vi "GUI_PR4000_flow.vi"() -> ()   [LabVIEW 2013]
uses:
  Shared/GUI_Template/GUI_master/tcp_new_data_event.ctl
  Shared/GUI_Template/GUI_master/tcp new data cluster.ctl
  controlFGV_TYPDEF.ctl
panel:
  in  "SlaveValue::1":dbl=25.5 caption="Slave value (%)" min=0.0 max=100.0 format="%_4f"
  in  "slaveenable::1":bool caption="Slave Mode"
  in  "Data.Channel 2::1":dbl=25.5 caption="PR4000 Pressure 2" min=0.0 max=1000.0 format="%_4f"
  out "Data.Channel 2::3":dbl=25.5 caption="PR4000 Flow 2" min=0.0 max=1000.0 format="%_4f"
  in  "Tab Control":enum32{"Chart", "Devices"}(tab)
  out "XY Graph":cluster{dbl[], dbl[]}[](graph)
  in  "Auto-scale horizontal range":bool caption="Force selected range"
  in  "Range graph3 (hours) 2":dbl=3.0 caption="Range (hours)"
  in  "Clear":bool
  in  "GUIdevice 2":string="BELLA_PDR2000"
  in  "GUIdevice 1":string="PL1-PresCtrl-Low1"
  in  "GUIdevice 3":string="PL1-PresCtrl-Low2"
  out "pressure2::2":dbl=25.5 caption="PDR pressure 2" min=-100.0 max=500.0 format="%_4f"
  out "Data.Channel 1::3":dbl=25.5 caption="PR4000 Flow 1" min=0.0 max=1000.0 format="%_4f"
  in  "Data.Channel 1::1":dbl=25.5 caption="PR4000 Pressure 1" min=0.0 max=1000.0 format="%_4f"
  out "pressure::2":dbl=25.5 caption="PDR Pressure 1" min=-100.0 max=500.0 format="%_4f"
  out "error IO 2":errorcluster
  in  "insert tag":bool=TRUE
  out "tcp data event":T1
  in  "stop":bool
  in  "UDP error message":string
  # "Plasma 1 capillary pressure & flow"
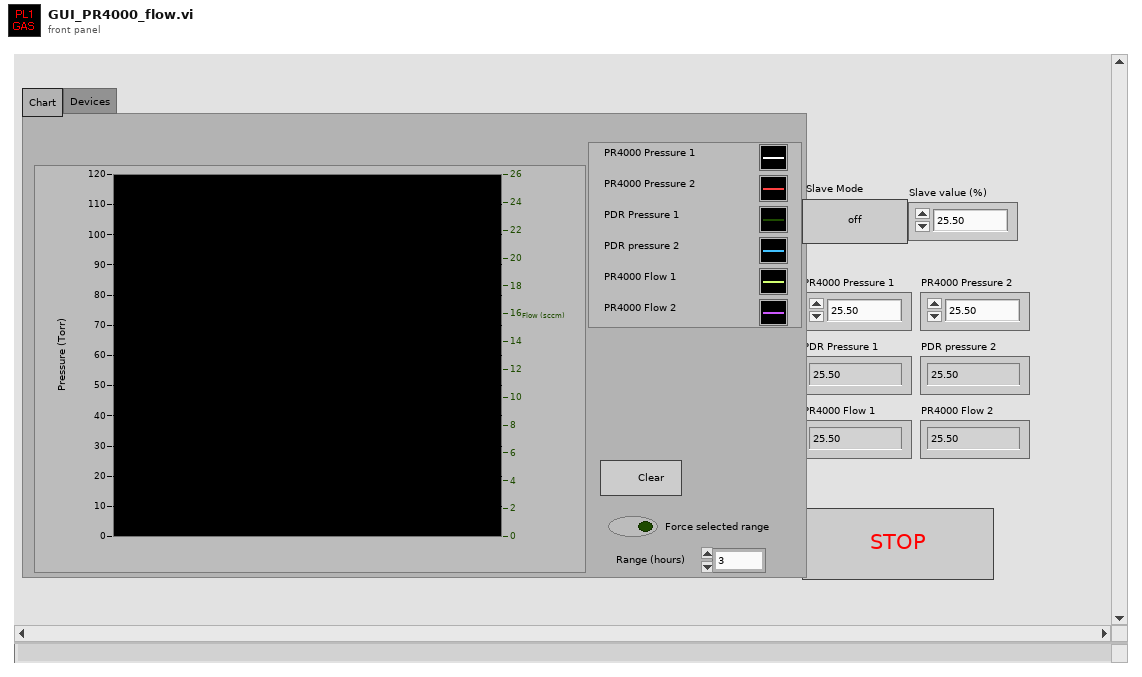
[diagram p1: front panel]
types:
  T1 = typedef "tcp_new_data_event.ctl" = refnum<user-event>
  T2 = typedef "tcp new data cluster.ctl" = cluster{"EventEnum":enum16{"new data", "connection status update"}, "Device name":string}
  T3 = typedef "controlFGV_TYPDEF.ctl" = enum16{"read", "write", "clear"}
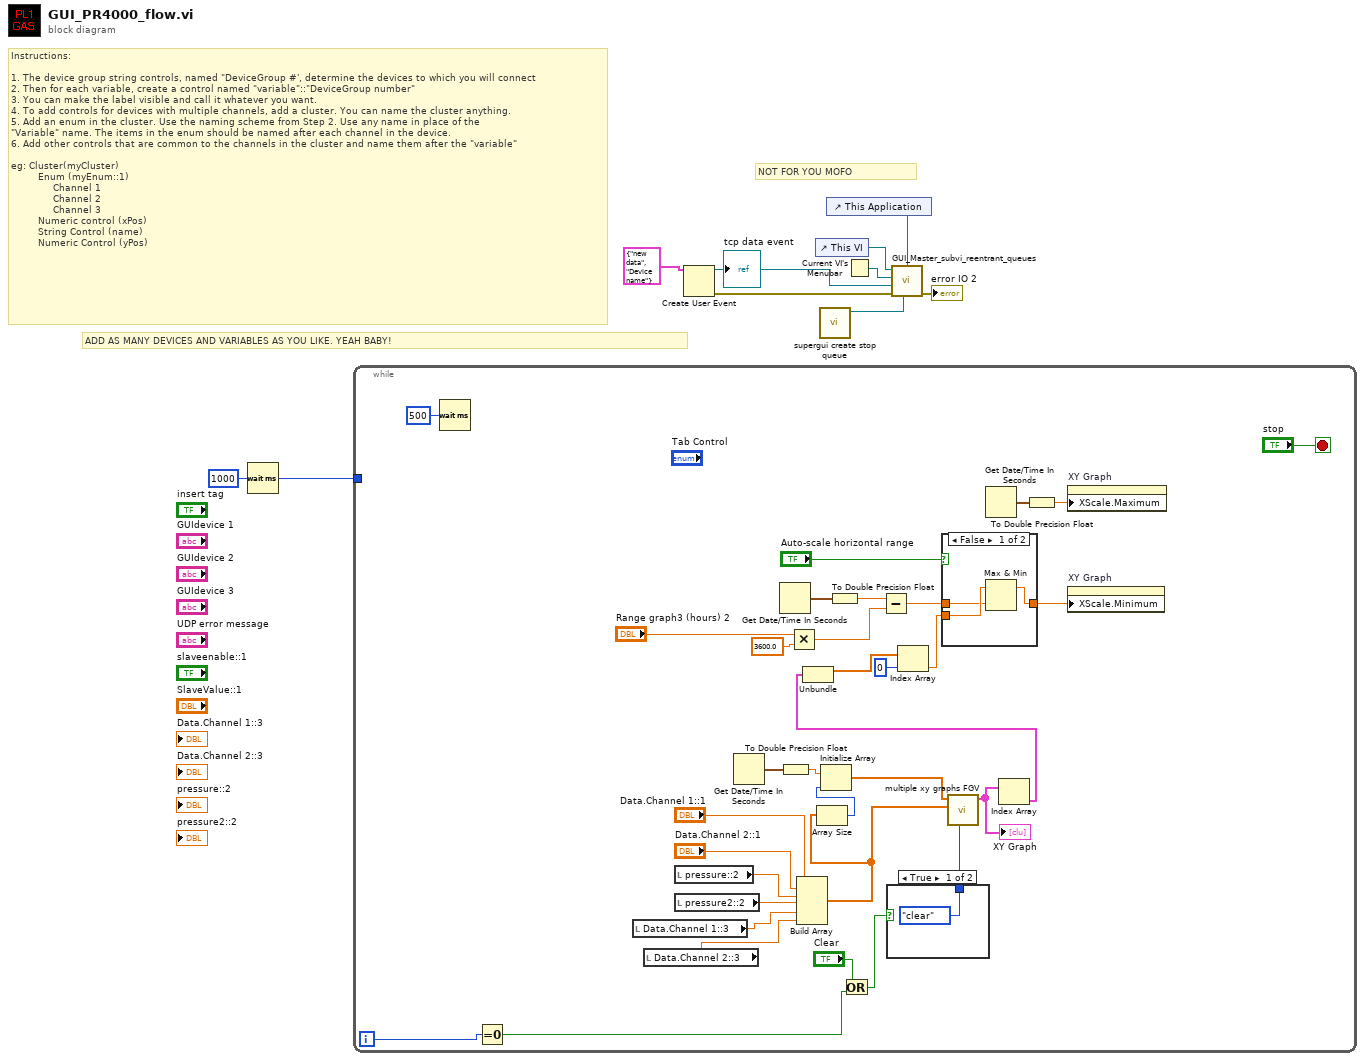
[diagram p0: block diagram]
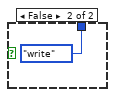
[diagram p2: hidden frame]
diagram:
  # "Instructions:\n\n1. The device group string controls, named \"DeviceGroup #', determine the devices to which you will connect\n2. Then for each variable, create a control named \"variable\"::\"DeviceGroup number\"\n3. You can make the label visible and call it whatever you want.\n4. To add controls for devices with multiple channels, add a cluster. You can name the cluster anything.\n5. Add an enum in the cluster. Use the naming scheme from Step 2. Use any name in place of the \n\"Variable\" name. The items in the enum should be named after each channel in the device. \n6. Add other controls that are common to the channels in the cluster and name them after the \"variable\"\n\neg: Cluster(myCluster)\n         Enum (myEnum::1)\n              Channel 1 \n              Channel 2\n              Channel 3\n         Numeric control (xPos)\n         String Control (name)\n         Numeric Control (yPos)"
  # "ADD AS MANY DEVICES AND VARIABLES AS YOU LIKE. YEAH BABY!"
  # "NOT FOR YOU MOFO"
  n1 = Wait (ms)(milliseconds to wait=u32 1000) -> (millisecond timer value=w3:u32)
  n2 = while {
    tunnel: w3 -> [_]
    i -> [w15]
    stop <- "stop" stop-if-true
    n3 = Wait (ms)(milliseconds to wait=u32 500) -> ()  [unwired: 1 out]
    n4 = Equal To 0?(x=w15) -> (x = 0?=w13:bool)
    n5 = local read "Data.Channel 1::3"() -> (w18:dbl)
    n6 = local read "Data.Channel 2::3"() -> (w17:dbl)
    n7 = local read "pressure::2"() -> (w27:dbl)
    n8 = local read "pressure2::2"() -> (w26:dbl)
    n9 = Get Date/Time In Seconds() -> (seconds since 1Jan1904=w25:timestamp)
    n10 = Get Date/Time In Seconds() -> (seconds since 1Jan1904=w37:timestamp)
    n11 = To Double Precision Float(number=w25) -> (double precision float=w24:dbl)
    n12 = Multiply(x="Range graph3 (hours) 2", y=3600.0) -> (x*y=w39:dbl)
    n13 = Build Array("Data.Channel 1::1", "Data.Channel 2::1", w27, w26, w18, w17) -> (w20:dbl[])
    n14 = Array Size(array=w20) -> (size(s)=w19:i32)
    n15 = Initialize Array(w24, w19) -> (w22:dbl[])
    n16 = To Double Precision Float(number=w37) -> (double precision float=w43:dbl)
    n17 = Or(x="Clear", y=w13) -> (x .or. y?=w12:bool)
    n18 = Subtract(x=w43, y=w39) -> (x-y=w41:dbl)
    n19 = case shown="True" w12 {
      tunnel: [controlFGV_TYPDEF."clear" ("command") controlFGV_TYPDEF."write" ("command")] -> w21
      frame True {
      }
      frame False {
      }
    }
    n20 = call "multiple xy graphs FGV.vi"("command"=w21, "Y values"=w20, "X values"=w22) -> ("XY Graph"=w23:cluster{dbl[], dbl[]}[])  [unwired: 8 in]
    "XY Graph" <- w23
    n21 = Get Date/Time In Seconds() -> (seconds since 1Jan1904=w33:timestamp)
    n22 = Index Array(array=w23) -> (element=w31:cluster{dbl[], dbl[]})  [unwired: 1 in]
    n23 = Unbundle(w31) -> (w30:dbl[])  [unwired: 1 out]
    n24 = Index Array(array=w30, index=0) -> (element=w35:dbl)
    n25 = case shown="False" "Auto-scale horizontal range" {
      tunnel: w35 -> [w47 _]
      tunnel: w41 -> [w46 w49]
      tunnel: [w48 w49] -> w34
      frame False {
        n26 = Max & Min(x=w47, y=w46) -> (max(x,y)=w48:dbl)  [unwired: 1 out]
      }
      frame True {
      }
    }
    n27 = To Double Precision Float(number=w33) -> (double precision float=w32:dbl)
    n28 = property on="XY Graph" class="XYGraph (strict)"("XScale.Maximum"=w32) -> ()  [unwired: 2 in, 2 out]
    n29 = property on="XY Graph" class="XYGraph (strict)"("XScale.Minimum"=w34) -> ()  [unwired: 2 in, 2 out]
  }
  n30 = Create User Event(user event datatype=T2 {"EventEnum"=enum."new data", "Device name"="Device name"} ("New Event")) -> (user event=w5:refnum<user-event>, error out=w10:errorcluster)  [unwired: 1 in]
  "tcp data event" <- w5
  n31 = control-ref of="This VI"() -> (w7:refnum<vi>)
  n32 = call "supergui create stop queue.vi"() -> ("STOP Queue out"=w1:refnum<queue>)  [unwired: 11 in]
  n33 = control-ref of="This Application"() -> (w4:refnum<vi>)
  n34 = Current VI's Menubar() -> (w8:refnum<k9>)
  n35 = call "GUI_Master_subvi_reentrant_queues.vi"("STOP Queue in"=w1, "This Application"=w4, "error in (no error)"=w10, "tcp data event"=w5, "Caller menu reference"=w8, "Caller VI ref"=w7) -> ("error out"=→"error IO 2":errorcluster)  [unwired: 5 in]
